vi "parametric-curve.vi"(7 "LabVIEW Web Service Request":refnum<class "Web Request.lvclass">) -> ()   [LabVIEW 2016]
uses:
  <vilib>/wsapi/Web Request.lvclass
  <vilib>/Analysis/6fits.llb/Prediction Interval (Gauss).vi
  <vilib>/Analysis/NI_AALPro.lvlib
panel:
  out "value":string
  # "Use the Web Service Request input terminal to call the VIs on the Web Services palette. Do not remove it from the connector pane unless you don't need access to the palette."
  # "Each additional control wired to the connector pane will be available as an input in the URL. To include an indicator in terminal-mode output (the default setting), it must also be wired to the connector pane."
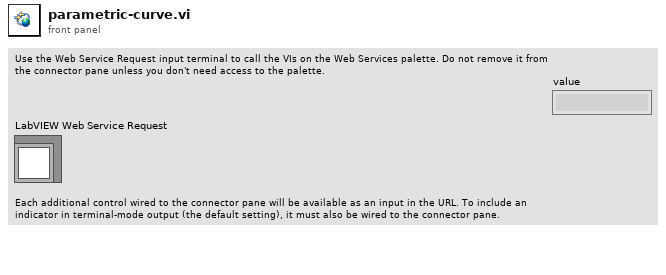
[diagram p1: front panel]
types:
  T1 = cluster{"X":dbl[], "Y":dbl[], "Best Gaussian Fit":dbl[], "Upper Bound":dbl[], "Lower Bound":dbl[]}
  T2 = enum16{"Linear", "Exponential", "Power", "Gaussian", "Logarithmic"}
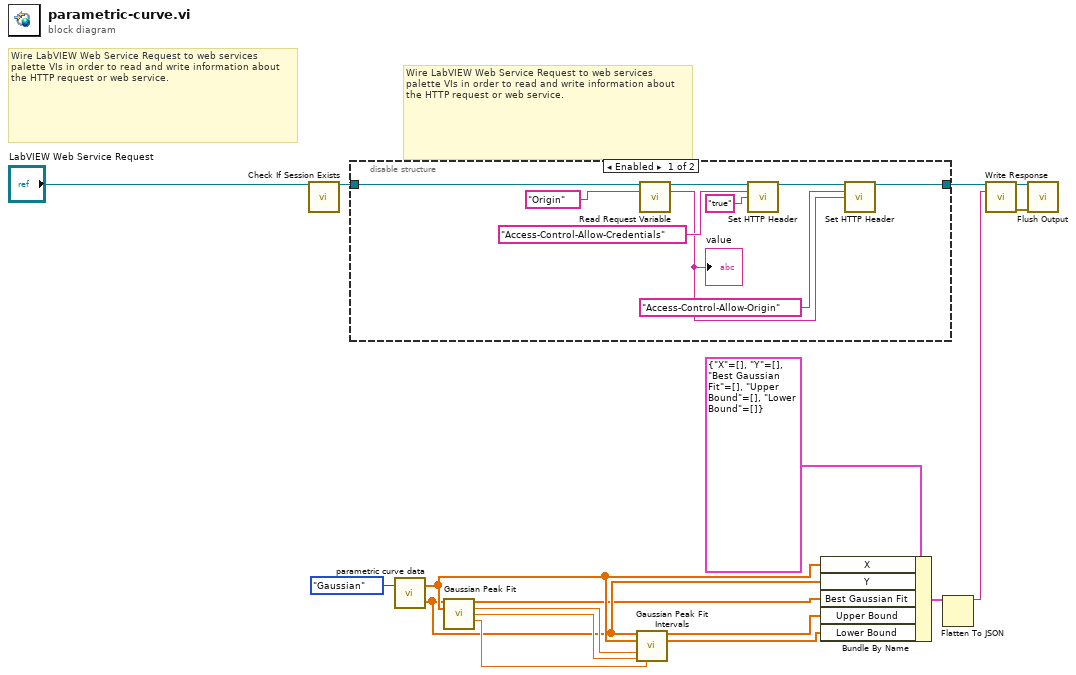
[diagram p0: block diagram]
diagram:
  # "Wire LabVIEW Web Service Request to web services palette VIs in order to read and write information about the HTTP request or web service."
  # "Wire LabVIEW Web Service Request to web services palette VIs in order to read and write information about the HTTP request or web service."
  n1 = call <vilib>:"Check If Session Exists.vi"("LabVIEW Web Service Request"="LabVIEW Web Service Request") -> ("LabVIEW Web Service Request out"=w3:refnum<class "Web Request.lvclass">)  [unwired: 12 in, 2 out]
  n2 = disable-structure shown="Enabled" {
    disable-tunnel: w3 -> [w22 w27]
    disable-tunnel: [w18 _] -> w1
    frame Enabled {
      n3 = call <vilib>:"Read Request Variable.vi"("LabVIEW Web Service Request"=w22, "variable name"="Origin") -> ("LabVIEW Web Service Request out"=w21:refnum<class "Web Request.lvclass">, "value"=w19:string)  [unwired: 11 in, 1 out]
      "value" <- w19
      n4 = call <vilib>:"Set HTTP Header.vi"("LabVIEW Web Service Request"=w21, "header"="Access-Control-Allow-Credentials", "header value"="true") -> ("LabVIEW Web Service Request out"=w25:refnum<class "Web Request.lvclass">)  [unwired: 11 in, 1 out]
      n5 = call <vilib>:"Set HTTP Header.vi"("LabVIEW Web Service Request"=w25, "header"="Access-Control-Allow-Origin", "header value"=w19) -> ("LabVIEW Web Service Request out"=w18:refnum<class "Web Request.lvclass">)  [unwired: 11 in, 1 out]
    }
    frame Disabled {
    }
  }
  n6 = call "parametric curve data.vi"("Signal type"=T2."Gaussian") -> ("Y"=w11:dbl[], "X"=w12:dbl[])  [unwired: 1 in]
  n7 = call <vilib>:"Gaussian Peak Fit.vi"("Y"=w11, "X"=w12) -> ("Best Gaussian Fit"=w10:dbl[], "amplitude"=w16:dbl, "center"=w15:dbl, "standard deviation"=w14:dbl)  [unwired: 7 in, 3 out]
  n8 = call-poly <vilib>:"Gaussian Peak Fit Intervals.vi"("Y"=w11, "X"=w12, "amplitude"=w16, "center"=w15, "standard deviation"=w14) -> ("Upper Bound"=w9:dbl[], "Lower Bound"=w8:dbl[])  [unwired: 8 in, 1 out]
  n9 = Bundle By Name(cluster=T1 {"X"=[], "Y"=[], "Best Gaussian Fit"=[], "Upper Bound"=[], "Lower Bound"=[]}, "X"=w12, "Y"=w11, "Best Gaussian Fit"=w10, "Upper Bound"=w9, "Lower Bound"=w8) -> (w13:T1)
  n10 = Flatten To JSON(anything=w13) -> (JSON string=w6:string)  [unwired: 2 in, 1 out]
  n11 = call <vilib>:"Write Response.vi"("LabVIEW Web Service Request"=w1, "response string"=w6) -> ("LabVIEW Web Service Request out"=w5:refnum<class "Web Request.lvclass">, "error out"=w4:errorcluster)  [unwired: 12 in]
  n12 = call <vilib>:"Flush Output.vi"("LabVIEW Web Service Request"=w5, "error in (no error)"=w4) -> ()  [unwired: 12 in, 2 out]
